vi "Convert JSONPath to Excel Table Path.vi"(8 "error in":errorcluster, 10 "Sheet Names":string[](array[string]), 11 "JSONPath":string) -> (0 "error out":errorcluster, 1 "Column":string, 2 "Row":i32, 3 "Table Name":string, 4 "Sub Object":string, 5 "Sheet Name":string)   [LabVIEW 2025, in "Config from Excel Table.lvclass"]
uses:
  Config from Excel Table.lvclass
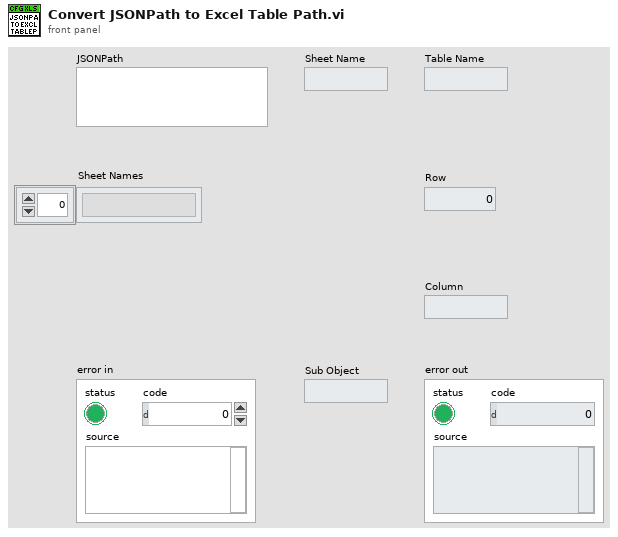
[diagram p1: front panel]
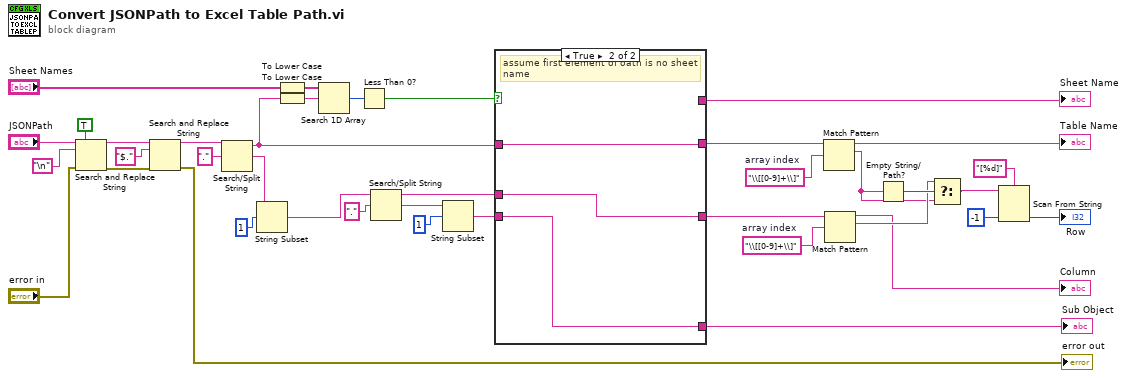
[diagram p0: block diagram]
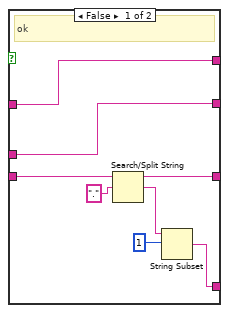
[diagram p2: hidden frame]
diagram:
  w17 = "\\[[0-9]+\\]"  # array index
  w19 = "\\[[0-9]+\\]"  # array index
  n1 = Search and Replace String(replace all?=TRUE ("replace all? (F)"), input string="JSONPath", search string="\n", error in="error in") -> (result string=w34:string, error out=w32:errorcluster)  [unwired: 4 in, 2 out]
  n2 = Search and Replace String(input string=w34, search string="$." ("search string/char (-)"), error in=w32) -> (result string=w29:string, error out=→"error out":errorcluster)  [unwired: 5 in, 2 out]
  n3 = Search/Split String(string=w29, search string/char (-)=".") -> (substring before match=w21:string, match + rest of string=w27:string)  [unwired: 1 in, 1 out]
  n4 = String Subset(string=w27, offset (0)=1) -> (substring=w26:string)  [unwired: 1 in]
  n5 = To Lower Case(string="Sheet Names") -> (all lower case string=w6:string[])
  n6 = To Lower Case(string=w21) -> (all lower case string=w5:string)
  n7 = Search 1D Array(1D array=w6, element=w5) -> (index of element=w23:i32)  [unwired: 1 in]
  n8 = Less Than 0?(x=w23) -> (x < 0?=w22:bool)
  n9 = Search/Split String(string=w26, search string/char (-)=".") -> (substring before match=w20:string, match + rest of string=w2:string)  [unwired: 1 in, 1 out]
  n10 = String Subset(string=w2, offset (0)=1) -> (substring=w1:string)  [unwired: 1 in]
  n11 = case shown="True" w22 {
    tunnel: w21 -> [w47 w50]
    tunnel: w20 -> [w46 w49]
    tunnel: [w46 w50] -> w8
    tunnel: [w47 _] -> w25
    tunnel: [w44 w49] -> w11
    tunnel: w1 -> [w40 w48]
    tunnel: [w41 w48] -> w4
    frame False {
      # "ok"
      n12 = Search/Split String(string=w40, search string/char (-)=".") -> (substring before match=w44:string, match + rest of string=w43:string)  [unwired: 1 in, 1 out]
      n13 = String Subset(string=w43, offset (0)=1) -> (substring=w41:string)  [unwired: 1 in]
    }
    frame True {
      # "assume first element of oath is no sheet name"
    }
  }
  "Sheet Name" <- w25
  "Sub Object" <- w4
  n14 = Match Pattern(string=w8, regular expression=w19) -> (before substring=→"Table Name":string, match substring=w13:string)  [unwired: 1 in, 2 out]
  n15 = Match Pattern(string=w11, regular expression=w17) -> (before substring=→"Column":string, match substring=w14:string)  [unwired: 1 in, 2 out]
  n16 = Empty String/Path?(string/path=w13) -> (empty?=w18:bool)
  n17 = Select(t=w14, s=w18, f=w13) -> (s? t:f=w12:string)
  n18 = Scan From String(format string="[%d]", input string=w12, default 1=-1 ("Row")) -> (output 1=→"Row":i32)  [unwired: 2 in, 3 out]
